vi "OutputCompressor.vi"   [LabVIEW 2020]
doc: "This VI sends commands to the compressor."
uses:
  f0d92a15-630b-4724-927c-98b746ccae8e.vi
  refnumbers.vi
  robotoutputs.vi
  driverdata.vi
  GRNF_Compressor.vi
types:
  T1 = typedef "WPI_CompressorDevRef.ctl" = cluster{"DevStatus":errorcluster, "Pneumatics Control Module":u8}
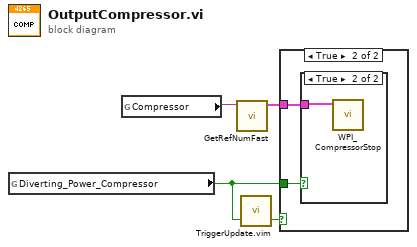
[diagram p0: block diagram]
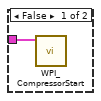
[diagram p3: hidden frame]
diagram:
  n1 = global read "robotoutputs.vi" "Diverting_Power_Compressor"() -> (w4:bool)
  n2 = global read "refnumbers.vi" "Compressor"() -> (w1:string)
  n3 = call-poly "GetRefNumFast.vi"("RefNum Name"=w1) -> ("Device Reference"=w2:T1)  [unwired: 5 in, 1 out]
  n4 = call "TriggerUpdate.vim"("Trigger"=w4) -> ("Update"=w3:bool)  [unwired: 2 in]
  n5 = case shown="True" w3 {
    tunnel: w4 -> [_ w6]
    tunnel: w2 -> [_ w5]
    frame False {
    }
    frame True {
      n6 = case shown="True" w6 {
        tunnel: w5 -> [w7 w8]
        frame False {
          n7 = call <vilib>:"WPI_CompressorStart.vi"("CompressorDevRef"=w7) -> ()  [unwired: 9 in, 2 out]
        }
        frame True {
          n8 = call <vilib>:"WPI_CompressorStop.vi"("CompressorDevRef"=w8) -> ()  [unwired: 9 in, 2 out]
        }
      }
    }
  }
